vi "Excel Demo-1.vi"() -> ()   [LabVIEW 2020]
doc: "Demo VI to generate data, write to Excel. Two columns of identifiers (Date, Time, Operator in one, Test, Humidity, Pressure in another) written first, then multiple rows of Time/Temperature data (one column for time, three columns for temperature).\n\nTables written to Excel are expected to be strings, while data plotted by Excel is expected to be numeric. We generate the Time/Temperature data as a 2D numeric array, saving a \"converted-to-string\" copy for the Data Table. Note that to plot the data, we need to transpose the array, with Time becoming the X values and Temperature(s) becoming the Y values.\n\nAfter writing the data to a new Excel spreadsheet, we save it in the same folder as this VI, using the name BS Demo.xlsx."
uses:
  <vilib>/addons/_office/excel.llb/Excel Easy Table (str).vi
  <vilib>/Utility/NIReport.llb/NI_report.lvclass
  <vilib>/addons/_office/NI_ReportGenerationToolkit.lvlib
  <vilib>/Utility/NIReport.llb/Excel/NI_Excel.lvclass
panel:
  in  "close report? (T)":bool=TRUE
  out "Error Out":errorcluster
  in  "Pressure":dbl=25.0
  in  "Humidity":dbl=30.0
  in  "Test":string="Temperature Demo"
  in  "Operator":string="LabVIEW Guru"
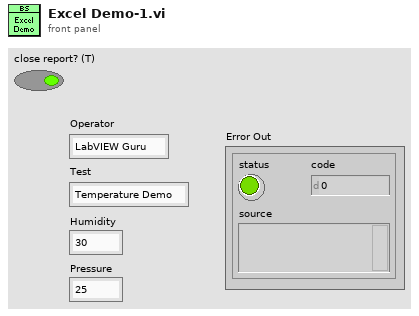
[diagram p1: front panel]
types:
  T1 = cluster{"left":i32, "top":i32, "height":dbl, "width":dbl}
  T2 = enum16{"Standard Report", "HTML", "Word", "Excel"}
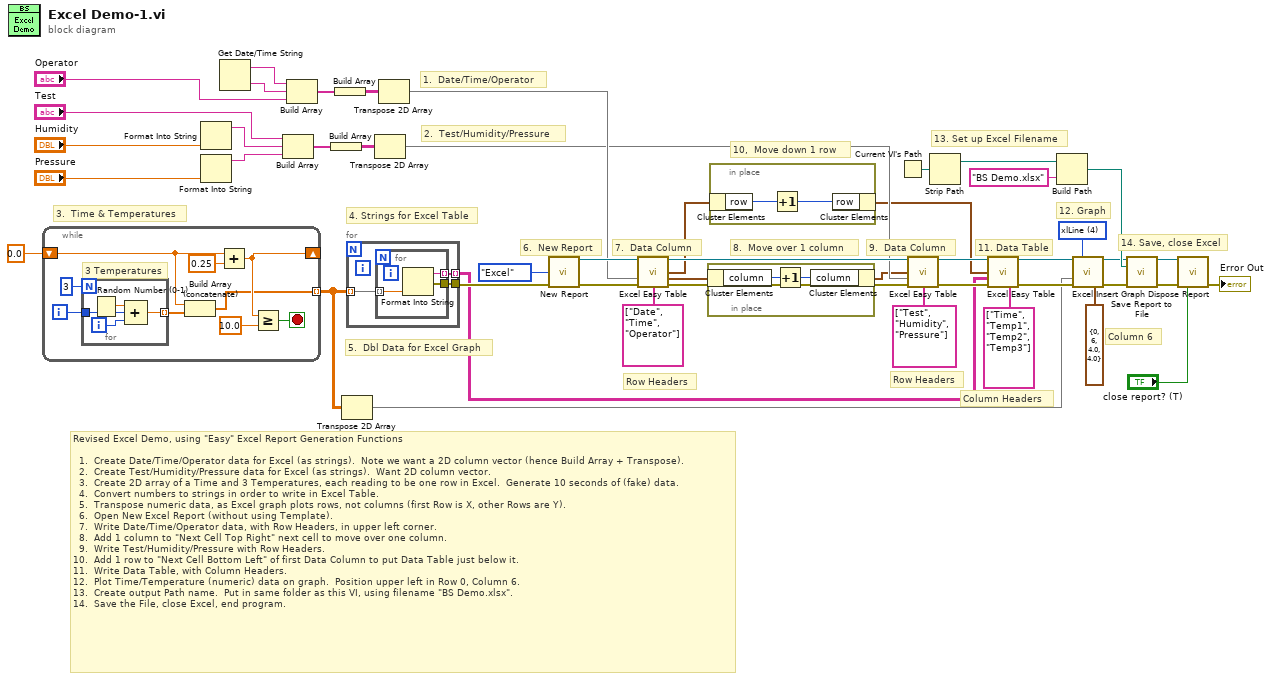
[diagram p0: block diagram]
diagram:
  w9 = 4 items=["xlColumnClustered"=51, "xlColumnStacked"=52, "xlColumnStacked100"=53, "xl3DColumnClustered"=54, "xl3DColumnStacked"=55, "xl3DColumnStacked100"=56, "xlBarClustered"=57, "xlBarStacked"=58, "xlBarStacked100"=59, "xl3DBarClustered"=60, "xl3DBarStacked"=61, "xl3DBarStacked100"=62, "xlLineStacked"=63, "xlLineStacked100"=64, "xlLineMarkers"=65, "xlLineMarkersStacked"=66, "xlLineMarkersStacked100"=67, "xlPieOfPie"=68, "xlPieExploded"=69, "xl3DPieExploded"=70, "xlBarOfPie"=71, "xlXYScatterSmooth"=72, "xlXYScatterSmoothNoMarkers"=73, "xlXYScatterLines"=74, "xlXYScatterLinesNoMarkers"=75, "xlAreaStacked"=76, "xlAreaStacked100"=77, "xl3DAreaStacked"=78, "xl3DAreaStacked100"=79, "xlDoughnutExploded"=80, "xlRadarMarkers"=81, "xlRadarFilled"=82, "xlSurface"=83, "xlSurfaceWireframe"=84, "xlSurfaceTopView"=85, "xlSurfaceTopViewWireframe"=86, "xlBubble"=15, "xlBubble3DEffect"=87, "xlStockHLC"=88, "xlStockOHLC"=89, "xlStockVHLC"=90, "xlStockVOHLC"=91, "xlCylinderColClustered"=92, "xlCylinderColStacked"=93, "xlCylinderColStacked100"=94, "xlCylinderBarClustered"=95, "xlCylinderBarStacked"=96, "xlCylinderBarStacked100"=97, "xlCylinderCol"=98, "xlConeColClustered"=99, "xlConeColStacked"=100, "xlConeColStacked100"=101, "xlConeBarClustered"=102, "xlConeBarStacked"=103, "xlConeBarStacked100"=104, "xlConeCol"=105, "xlPyramidColClustered"=106, "xlPyramidColStacked"=107, "xlPyramidColStacked100"=108, "xlPyramidBarClustered"=109, "xlPyramidBarStacked"=110, "xlPyramidBarStacked100"=111, "xlPyramidCol"=112, "xl3DColumn"=-4100, "xlLine"=4, "xl3DLine"=-4101, "xl3DPie"=-4102, "xlPie"=5, "xlXYScatter"=-4169, "xl3DArea"=-4098, "xlArea"=1, "xlDoughnut"=-4120, "xlRadar"=-4151] ("graph type (col clustered)")
  # "Column Headers"
  # "Revised Excel Demo, using \"Easy\" Excel Report Generation Functions\n\n  1.  Create Date/Time/Operator data for Excel (as strings).  Note we want a 2D column vector (hence Build Array + Transpose).\n  2.  Create Test/Humidity/Pressure data for Excel (as strings).  Want 2D column vector.\n  3.  Create 2D array of a Time and 3 Temperatures, each reading to be one row in Excel.  Generate 10 seconds of (fake) data.\n  4.  Convert numbers to strings in order to write in Excel Table.\n  5.  Transpose numeric data, as Excel graph plots rows, not columns (first Row is X, other Rows are Y).\n  6.  Open New Excel Report (without using Template).\n  7.  Write Date/Time/Operator data, with Row Headers, in upper left corner.\n  8.  Add 1 column to \"Next Cell Top Right\" next cell to move over one column.\n  9.  Write Test/Humidity/Pressure with Row Headers.\n10.  Add 1 row to \"Next Cell Bottom Left\" of first Data Column to put Data Table just below it.\n11.  Write Data Table, with Column Headers.\n12.  Plot Time/Temperature (numeric) data on graph.  Position upper left in Row 0, Column 6.\n13.  Create output Path name.  Put in same folder as this VI, using filename \"BS Demo.xlsx\".\n14.  Save the File, close Excel, end program."
  # "4. Strings for Excel Table"
  # "3.  Time & Temperatures"
  # "14. Save, close Excel"
  # "13. Set up Excel Filename"
  # "Column 6"
  # "12. Graph"
  # "11. Data Table"
  # "10,  Move down 1 row"
  # "9.  Data Column"
  # "8.  Move over 1 column"
  # "7.  Data Column"
  # "6.  New Report"
  # "5.  Dbl Data for Excel Graph"
  # "Row Headers"
  # "Row Headers"
  # "2.  Test/Humidity/Pressure"
  # "1.  Date/Time/Operator"
  n1 = while {
    shift-right: [w52] -> _
    shift-left: 0.0 -> [w53]
    tunnel: [w49] -> w5 mode=indexing
    i -> [w56]
    stop <- w50 stop-if-true
    # "3 Temperatures"
    n2 = for {
      N: 3 -> [_]
      tunnel: w56 -> [w59]
      tunnel: [w57] -> w54 mode=indexing
      i -> [w60]
      n3 = Random Number (0-1)() -> (number: 0 to 1=w58:dbl)
      n4 = Compound Arithmetic op=ADD(w58, w59, w60) -> (w57:dbl)
    }
    n5 = Build Array (concatenate)(w53, w54) -> (w49:dbl[])
    n6 = Add(x=w53, y=0.25) -> (x+y=w52:dbl)
    n7 = Greater Or Equal?(x=w52, y=10.0) -> (x >= y?=w50:bool)
  }
  n8 = Format Into String("Humidity") -> (resulting string=w34:string)  [unwired: 3 in, 1 out]
  n9 = Format Into String("Pressure") -> (resulting string=w33:string)  [unwired: 3 in, 1 out]
  n10 = Get Date/Time String() -> (date string=w47:string, time string=w46:string)  [unwired: 3 in]
  n11 = Build Array("Test", w34, w33) -> (w35:string[])
  n12 = Build Array(w47, w46, "Operator") -> (w44:string[])
  n13 = Build Array(w35) -> (w36:string[][])
  n14 = Build Array(w44) -> (w43:string[][])
  n15 = Transpose 2D Array(2D array=w5) -> (transposed array=w10:dbl[][])
  n16 = for {
    tunnel: w5 -> [w63] mode=indexing
    tunnel: [w62] -> w2 mode=indexing
    tunnel: [w61] -> w4
    n17 = for {
      tunnel: w63 -> [w66] mode=indexing
      tunnel: [w65] -> w62 mode=indexing
      tunnel: [w64] -> w61
      n18 = Format Into String(w66) -> (resulting string=w65:string, error out=w64:errorcluster)  [unwired: 3 in]
    }
  }
  n19 = Transpose 2D Array(2D array=w36) -> (transposed array=w27:string[][])
  n20 = Transpose 2D Array(2D array=w43) -> (transposed array=w40:string[][])
  n21 = call <vilib>:"New Report.vi"("report type"=T2."Excel", "error in (no error)"=w4) -> ("report out"=w41:refnum<class "NI_report.lvclass">, "error out"=w3:errorcluster)  [unwired: 12 in]
  n22 = call-poly <vilib>:"Excel Easy Table.vi"("report in"=w41, "text data"=w40, "error in (no error)"=w3, "row headers"=string[] ["Date", "Time", "Operator"] ("column headers")) -> ("report out"=w30:refnum<class "NI_report.lvclass">, "next cell bottom-left"=w23:cluster{"row":i32, "column":i32}, "next cell top-right"=w39:cluster{"row":i32, "column":i32}, "error out"=w31:errorcluster)  [unwired: 7 in, 1 out]
  n23 = in-place {
    n24 = in-place-cluster #1(w39) -> ("column"=w68:i32)
    n25 = Increment(x=w68) -> (x+1=w67:i32)
    n26 = in-place-cluster #1("column"=w67) -> (w21:cluster{"row":i32, "column":i32})
  }
  n27 = in-place {
    n28 = in-place-cluster #2(w23) -> ("row"=w70:i32)
    n29 = Increment(x=w70) -> (x+1=w69:i32)
    n30 = in-place-cluster #2("row"=w69) -> (w22:cluster{"row":i32, "column":i32})
  }
  n31 = Current VI's Path() -> (path=w20:path)
  n32 = call-poly <vilib>:"Excel Easy Table.vi"("report in"=w30, "start (0, 0)"=w21, "text data"=w27, "error in (no error)"=w31, "row headers"=string[] ["Test", "Humidity", "Pressure"] ("column headers")) -> ("report out"=w25:refnum<class "NI_report.lvclass">, "error out"=w26:errorcluster)  [unwired: 6 in, 3 out]
  n33 = Strip Path(path=w20) -> (stripped path=w19:path)  [unwired: 1 out]
  n34 = call-poly <vilib>:"Excel Easy Table.vi"("report in"=w25, "start (0, 0)"=w22, "text data"=w2, "error in (no error)"=w26, "column headers"=string[] ["Time", "Temp1", "Temp2", "Temp3"]) -> ("report out"=w14:refnum<class "NI_report.lvclass">, "error out"=w13:errorcluster)  [unwired: 6 in, 3 out]
  n35 = Build Path(base path=w19, name or relative path="BS Demo.xlsx") -> (appended path=w17:path)
  n36 = call <vilib>:"Excel Insert Graph.vi"("report in"=w14, "graph type (col clustered)"=w9, "data"=w10, "error in (no error)"=w13, "position/size"=T1 {"left"=0, "top"=6, "height"=4.0, "width"=4.0}) -> ("report out"=w11:refnum<class "NI_report.lvclass">, "error out"=w12:errorcluster)  [unwired: 9 in]
  n37 = call-dynamic "Save Report to File.vi"("report in"=w11, "report file path"=w17, "error in (no error)"=w12) -> ("report out"=w16:refnum<class "NI_report.lvclass">, "error out"=w15:errorcluster)  [unwired: 11 in]
  n38 = call-dynamic "Dispose Report.vi"("report in"=w16, "error in (no error)"=w15, "close report? (T)"="close report? (T)") -> ("error out"=→"Error Out":errorcluster)  [unwired: 12 in]
